vi "First1Second1glb.vi"() -> ()   [LabVIEW 2020]
panel:
  in  "stop":bool
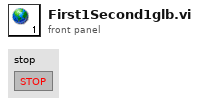
[diagram p1: front panel]
diagram:
